vi "Start.vi"(8 "Error In":errorcluster, 11 "AutoData":T1) -> (0 "Error Out":errorcluster, 3 "AutoData out":T1)   [LabVIEW 2019, in "AutoMode.lvlib"]
uses:
  AutoMode.lvlib
  Cluster - AutoModeData.ctl
  MainController/Cluster - TestSettings.ctl
  MainController/Cluster - HardwareConfiguration.ctl
  MainController/Cluster - TestResults.ctl
  Cluster - AutoModeMessage.ctl
  Enum - AutoModeState.ctl
  MainController/Cluster - MainControllerMessage.ctl
  MainController/Enum - MainState.ctl
  Utilites/Utilities.lvlib
  MainController/MainController.lvlib
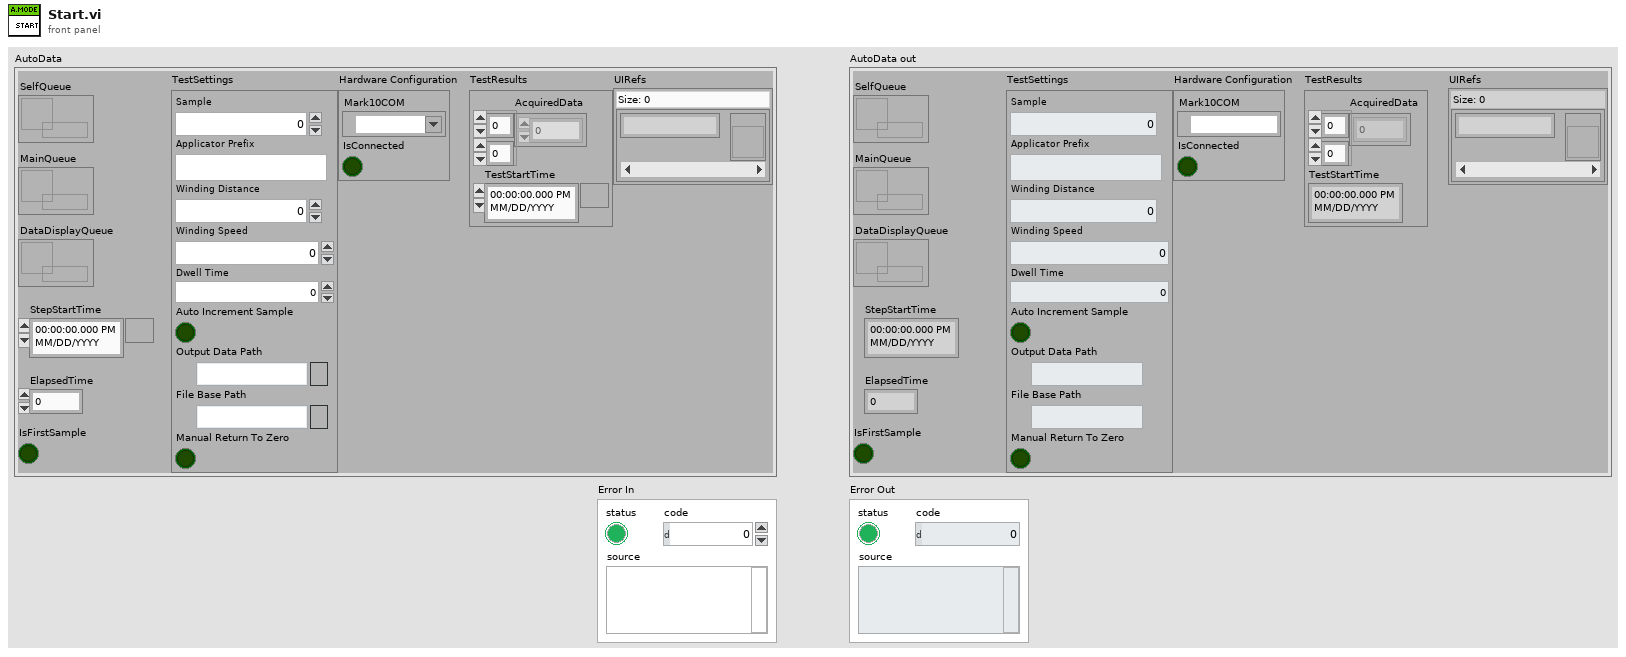
[diagram p1: front panel]
types:
  T1 = typedef "AutoMode.lvlib/Cluster - AutoModeData.ctl" = cluster{"DataDisplayQueue":refnum<queue>, "StepStartTime":timestamp, "TestSettings":T2, "Hardware Configuration":T3, "TestResults":T4, "ElapsedTime":dbl, "IsFirstSample":bool, "UIRefs":map{string, refnum<vi>}, "SelfQueue":refnum<queue>, "MainQueue":refnum<queue>}
  T2 = typedef "MainController.lvlib/Cluster - TestSettings.ctl" = cluster{"Sample":u32, "Applicator Prefix":string, "Winding Distance":dbl, "Winding Speed":dbl, "Dwell Time":dbl, "Auto Increment Sample":bool, "Output Data Path":path, "File Base Path":path, "Manual Return To Zero":bool}
  T3 = typedef "MainController.lvlib/Cluster - HardwareConfiguration.ctl" = cluster{"Mark10COM":refnum<visa-resource-name>, "IsConnected":bool}
  T4 = typedef "MainController.lvlib/Cluster - TestResults.ctl" = cluster{"AcquiredData":dbl[][], "TestStartTime":timestamp}
  T5 = typedef "AutoMode.lvlib/Enum - AutoModeState.ctl" = enum16{"Initialize", "Idle", "UpdateConfig", "UpdateHWConfig", "BroadcastSettings", "Start", "CheckValidReportPath", "Winding", "WaitForWinding", "Unwind", "WaitForUnwind", "Stop", "Abort", "WriteDataToFile", "EventTriggered", "GenerateFilePath", "ZeroPosition", "GotoZero", "Error", "Exit"}
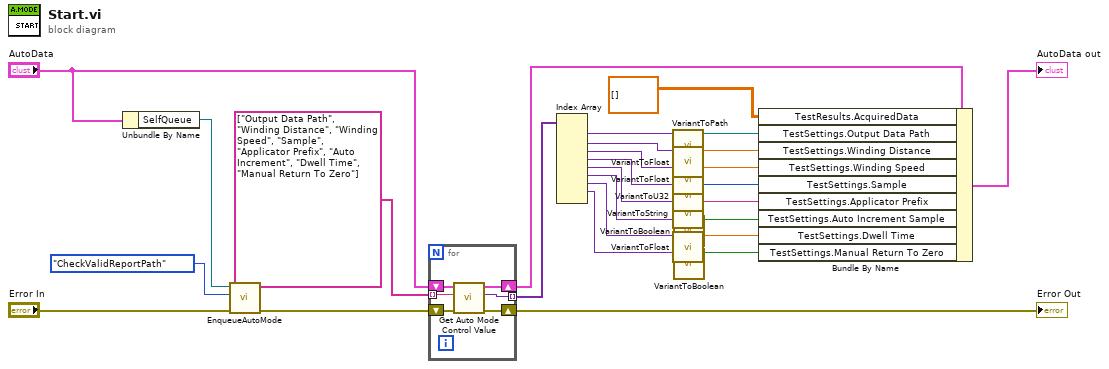
[diagram p0: block diagram]
diagram:
  n1 = Unbundle By Name("AutoData") -> ("SelfQueue"=w24:refnum<queue>)
  n2 = call "EnqueueAutoMode.vi"("error in (no error)"="Error In", "AutoState"=Enum_-_AutoModeState."CheckValidReportPath" ("CycleTestState"), "Queue in"=w24) -> ("error out"=w25:errorcluster)  [unwired: 7 in, 1 out]
  n3 = for {
    tunnel: string[] ["Output Data Path", "Winding Distance", "Winding Speed", "Sample", "Applicator Prefix", "Auto Increment", "Dwell Time", "Manual Return To Zero"] ("key") -> [w30] mode=indexing
    shift-right: [w32] -> w21
    shift-left: w25 -> [w33]
    shift-right: [w29] -> w19
    shift-left: "AutoData" -> [w31]
    tunnel: [w28] -> w17 mode=indexing
    n4 = call "Get Auto Mode Control Value.vi"("Error In"=w33, "key"=w30, "AutoData"=w31) -> ("Error Out"=w32:errorcluster, "Value"=w28:variant, "AutoData out"=w29:T1)  [unwired: 6 in]
  }
  "Error Out" <- w21
  n5 = Index Array(array=w17) -> (element #1=w16:variant, element #2=w15:variant, element #3=w14:variant, element #4=w13:variant, element #5=w9:variant, element #6=w5:variant, element #7=w7:variant, element #8=w2:variant)  [unwired: 9 in, 1 out]
  n6 = call "VariantToPath.vi"("Variant"=w16) -> ("Value"=w1:path)  [unwired: 9 in, 1 out]
  n7 = call "VariantToFloat.vi"("Variant"=w15) -> ("Value"=w12:dbl)  [unwired: 9 in, 1 out]
  n8 = call "VariantToFloat.vi"("Variant"=w14) -> ("Value"=w11:dbl)  [unwired: 9 in, 1 out]
  n9 = call "VariantToU32.vi"("Variant"=w13) -> ("Value"=w10:u32)  [unwired: 9 in, 1 out]
  n10 = call "VariantToString.vi"("Variant"=w9) -> ("Value"=w8:string)  [unwired: 9 in, 1 out]
  n11 = call "VariantToFloat.vi"("Variant"=w7) -> ("Value"=w6:dbl)  [unwired: 9 in, 1 out]
  n12 = call "VariantToBoolean.vi"("Variant"=w5) -> ("Value"=w4:bool)  [unwired: 9 in, 1 out]
  n13 = call "VariantToBoolean.vi"("Variant"=w2) -> ("Value"=w3:bool)  [unwired: 9 in, 1 out]
  n14 = Bundle By Name(cluster=w19, "TestResults.AcquiredData"=dbl[][] [], "TestSettings.Output Data Path"=w1, "TestSettings.Winding Distance"=w12, "TestSettings.Winding Speed"=w11, "TestSettings.Sample"=w10, "TestSettings.Applicator Prefix"=w8, "TestSettings.Auto Increment Sample"=w4, "TestSettings.Dwell Time"=w6, "TestSettings.Manual Return To Zero"=w3) -> (→"AutoData out":T1)
